vi "Read ILC DAC Settings.vi"(8 "error in (no error)":errorcluster, 11 "Boot Loader in":refnum<class "Boot Loader.lvclass">) -> (0 "error out":errorcluster, 2 "ILC ADC Settings":T1={"Voltage Reference"=4.096, "Min Counts"=0, "Max Counts"=65535} {"Voltage Reference" format="%.3f"}, 3 "Boot Loader out":refnum<class "Boot Loader.lvclass">)   [LabVIEW 2015, in "Boot Loader.lvclass"]
uses:
  Boot Loader.lvclass
  <userlib>/Common/ILC/Typedefs/DAC Settings.ctl
  Settings/Settings.lvclass
  <userlib>/Common/ILC/Typedefs/ILCTypedefs.lvlib
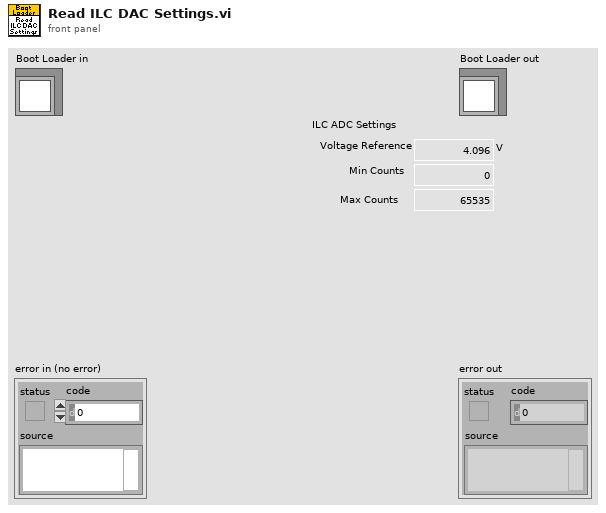
[diagram p1: front panel]
types:
  T1 = typedef "ILCCommon.lvlib/ILCTypedefs.lvlib/DAC Settings.ctl" = cluster{"Voltage Reference":dbl[unit], "Min Counts":i32, "Max Counts":i32}
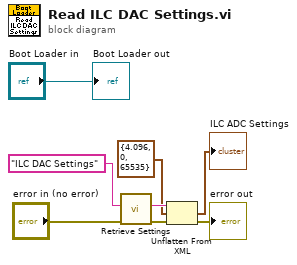
[diagram p0: block diagram]
diagram:
  n1 = call "Retrieve Settings.vi"("error in (no error)"="error in (no error)", "configName"="ILC DAC Settings") -> ("error out"=w7:errorcluster, "xmlConfig"=w5:string)  [unwired: 7 in, 1 out]
  n2 = Unflatten From XML(xml string=w5, type=T1 {"Voltage Reference"=4.096, "Min Counts"=0, "Max Counts"=65535} ("DAC Settings"), error in (no error)=w7) -> (value=→"ILC ADC Settings":T1, error out=→"error out":errorcluster)
  "Boot Loader out" <- "Boot Loader in"
